vi "xmltddresult.vi"(8 "second result":string, 9 "TDD spec":string, 10 "TX data":string[](array[string]), 11 "RX data":string[](array[string])) -> (2 "TX array":string[](array[string]), 3 "RX array":string[](array[string]))   [LabVIEW 2011]
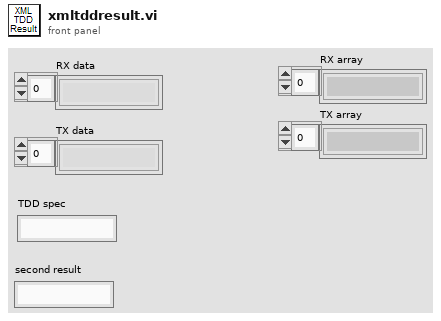
[diagram p1: front panel]
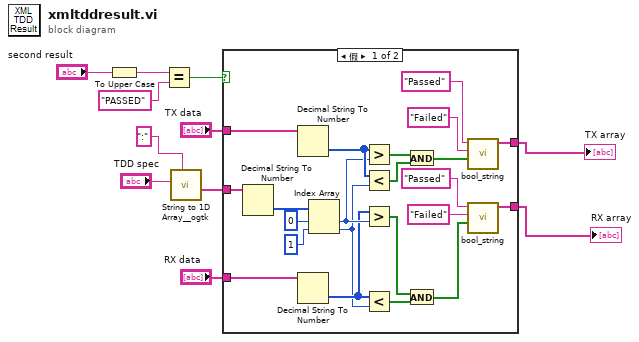
[diagram p0: block diagram]
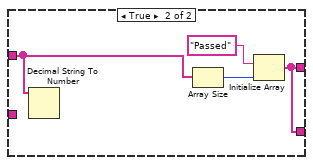
[diagram p2: hidden frame]
diagram:
  n1 = To Upper Case(1:"second result") -> (0:w10:string)
  n2 = Equal?(x=w10, y="PASSED") -> (x = y?=w8:bool)
  n3 = call <userlib>:"String to 1D Array__ogtk.vi"("delimiter (Tab)"=":", "string"="TDD spec") -> ("Array of Strings"=w3:string[])  [unwired: 9 in]
  n4 = case shown="假" w8 {
    tunnel: "TX data" -> [w33 w35]
    tunnel: [w29 w34] -> w2
    tunnel: [w26 w34] -> w1
    tunnel: "RX data" -> [w32 _]
    tunnel: w3 -> [w25 _]
    frame False {
      n5 = Decimal String To Number(string=w25) -> (number=w24:i32[])  [unwired: 2 in, 1 out]
      n6 = Decimal String To Number(string=w33) -> (number=w21:i32[])  [unwired: 2 in, 1 out]
      n7 = Decimal String To Number(string=w32) -> (number=w16:i32[])  [unwired: 2 in, 1 out]
      n8 = Index Array(array=w24, index #1=0 ("索引"), index #2=1 ("索引")) -> (element #1=w17:i32, element #2=w15:i32)
      n9 = Greater?(x=w21, y=w17) -> (0:w20:bool[])
      n10 = Less?(x=w21, y=w15) -> (x < y?=w19:bool[])
      n11 = Greater?(x=w16, y=w17) -> (0:w14:bool[])
      n12 = Less?(x=w16, y=w15) -> (x < y?=w13:bool[])
      n13 = And(x=w20, y=w19) -> (x .and. y?=w18:bool[])
      n14 = And(x=w14, y=w13) -> (x .and. y?=w12:bool[])
      n15 = call "bool_string.vi"("boolean array"=w18, "FalseValue"="Failed", "TrueValue"="Passed") -> ("string array"=w29:string[])  [unwired: 8 in]
      n16 = call "bool_string.vi"("boolean array"=w12, "FalseValue"="Failed", "TrueValue"="Passed") -> ("string array"=w26:string[])  [unwired: 8 in]
    }
    frame True {
      n17 = Decimal String To Number(string=w35) -> ()  [unwired: 2 in, 2 out]
      n18 = Array Size(array=w35) -> (size(s)=w36:i32)
      n19 = Initialize Array("Passed" ("y"), w36) -> (w34:string[])
    }
  }
  "RX array" <- w1
  "TX array" <- w2
